vi "ActiveX - StringArray2WordTables.vi"(8 "error in (no error)":errorcluster caption="错误输入（无错误）", 10 "文件存储路径":path=path "C:/WorkSpace/LabVIEW/ActiveX StrArr2WordTables/Test.docx", 11 "文本数组":string[][](array[string])=[["1", "2"], ["3", "4"]]) -> (0 "error out":errorcluster caption="错误输出")   [LabVIEW 2019]
uses:
  <vilib>/Utility/NIReport.llb/Report Type.ctl
  <vilib>/Utility/NIReport.llb/Append Text Table to Report (wrap).vi
  <vilib>/Utility/NIReport.llb/NI_report.lvclass
  <vilib>/Utility/NIReport.llb/NI_ReportGenerationCore.lvlib
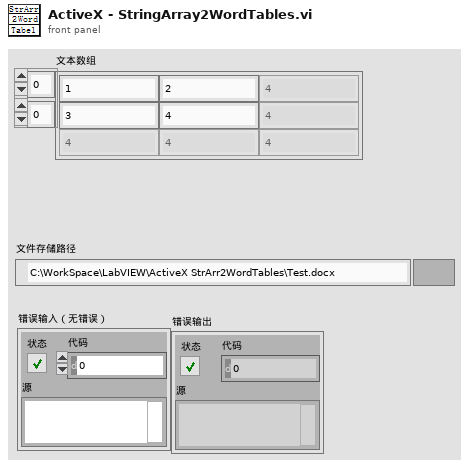
[diagram p1: front panel]
types:
  T1 = typedef "NI_ReportGenerationCore.lvlib/Report Type.ctl" = enum16{"HTML", "Word", "Excel"}
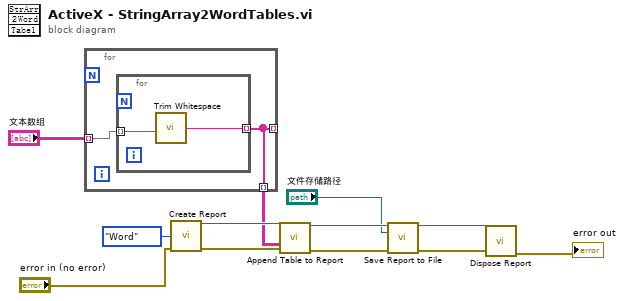
[diagram p0: block diagram]
diagram:
  n1 = for {
    tunnel: "文本数组" -> [w14] mode=indexing
    tunnel: [w13] -> _ mode=indexing
    tunnel: [w13] -> w1 mode=indexing
    n2 = for {
      tunnel: w14 -> [w16] mode=indexing
      tunnel: [w15] -> w13 mode=indexing
      n3 = call <vilib>:"Trim Whitespace.vi"("string"=w16) -> ("trimmed string"=w15:string)  [unwired: 1 in]
    }
  }
  n4 = call <vilib>:"Create Report.vi"("report type"=Report_Type."Word", "error in (no error)"="error in (no error)") -> ("report out"=w11:refnum<class "NI_report.lvclass">, "error out"=w10:errorcluster)  [unwired: 12 in]
  n5 = call-poly <vilib>:"Append Table to Report.vi"("report in"=w11, "text data"=w1, "error in (no error)"=w10) -> ("report out"=w9:refnum<class "NI_report.lvclass">, "error out"=w8:errorcluster)  [unwired: 9 in, 2 out]
  n6 = call-dynamic "Save Report to File.vi"("report in"=w9, "report file path"="文件存储路径", "error in (no error)"=w8) -> ("report out"=w6:refnum<class "NI_report.lvclass">, "error out"=w5:errorcluster)  [unwired: 11 in]
  n7 = call-dynamic "Dispose Report.vi"("report in"=w6, "error in (no error)"=w5) -> ("error out"=→"error out":errorcluster)  [unwired: 13 in]
